vi "Door.vi"() -> ()   [LabVIEW 2011]
uses:
  <vilib>/LabVIEW Interface for Arduino/Type Defs/Board Type.ctl
  <vilib>/LabVIEW Interface for Arduino/Type Defs/Pin Mode.ctl
  <vilib>/LabVIEW Interface for Arduino/LabVIEW Interface for Arduino.lvlib
panel:
  in  "stop 13":bool
  out "Voltage 4":dbl(knob) scale=0.0..5.0
  out "Key Switch open":bool
  out "Numeric":i32
  out "Numeric 2":i32
  out "Door Open":bool
  out "Door Close":bool
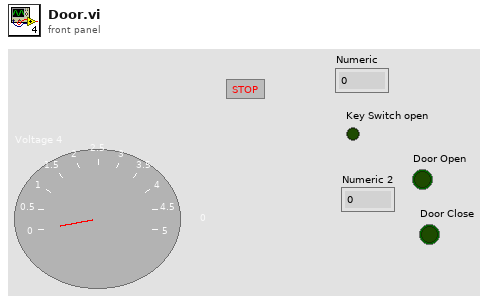
[diagram p1: front panel]
types:
  T1 = typedef "LabVIEW Interface for Arduino.lvlib/Board Type.ctl" = enum16{"Uno", "Dimuelanove w/Atmega 328", "Mega 2560"}
  T2 = typedef "LabVIEW Interface for Arduino.lvlib/Pin Mode.ctl" = enum8{"Input", "Output"}
  T3 = typedef "LabVIEW Interface for Arduino.lvlib/Arduino Resource.ctl" = cluster{"VISA resource":refnum<visa-resource-name>, "Board Type":T1, "Connection Type":enum8{"USB / Serial"}, "Bytes Per Packet (15)":u8}
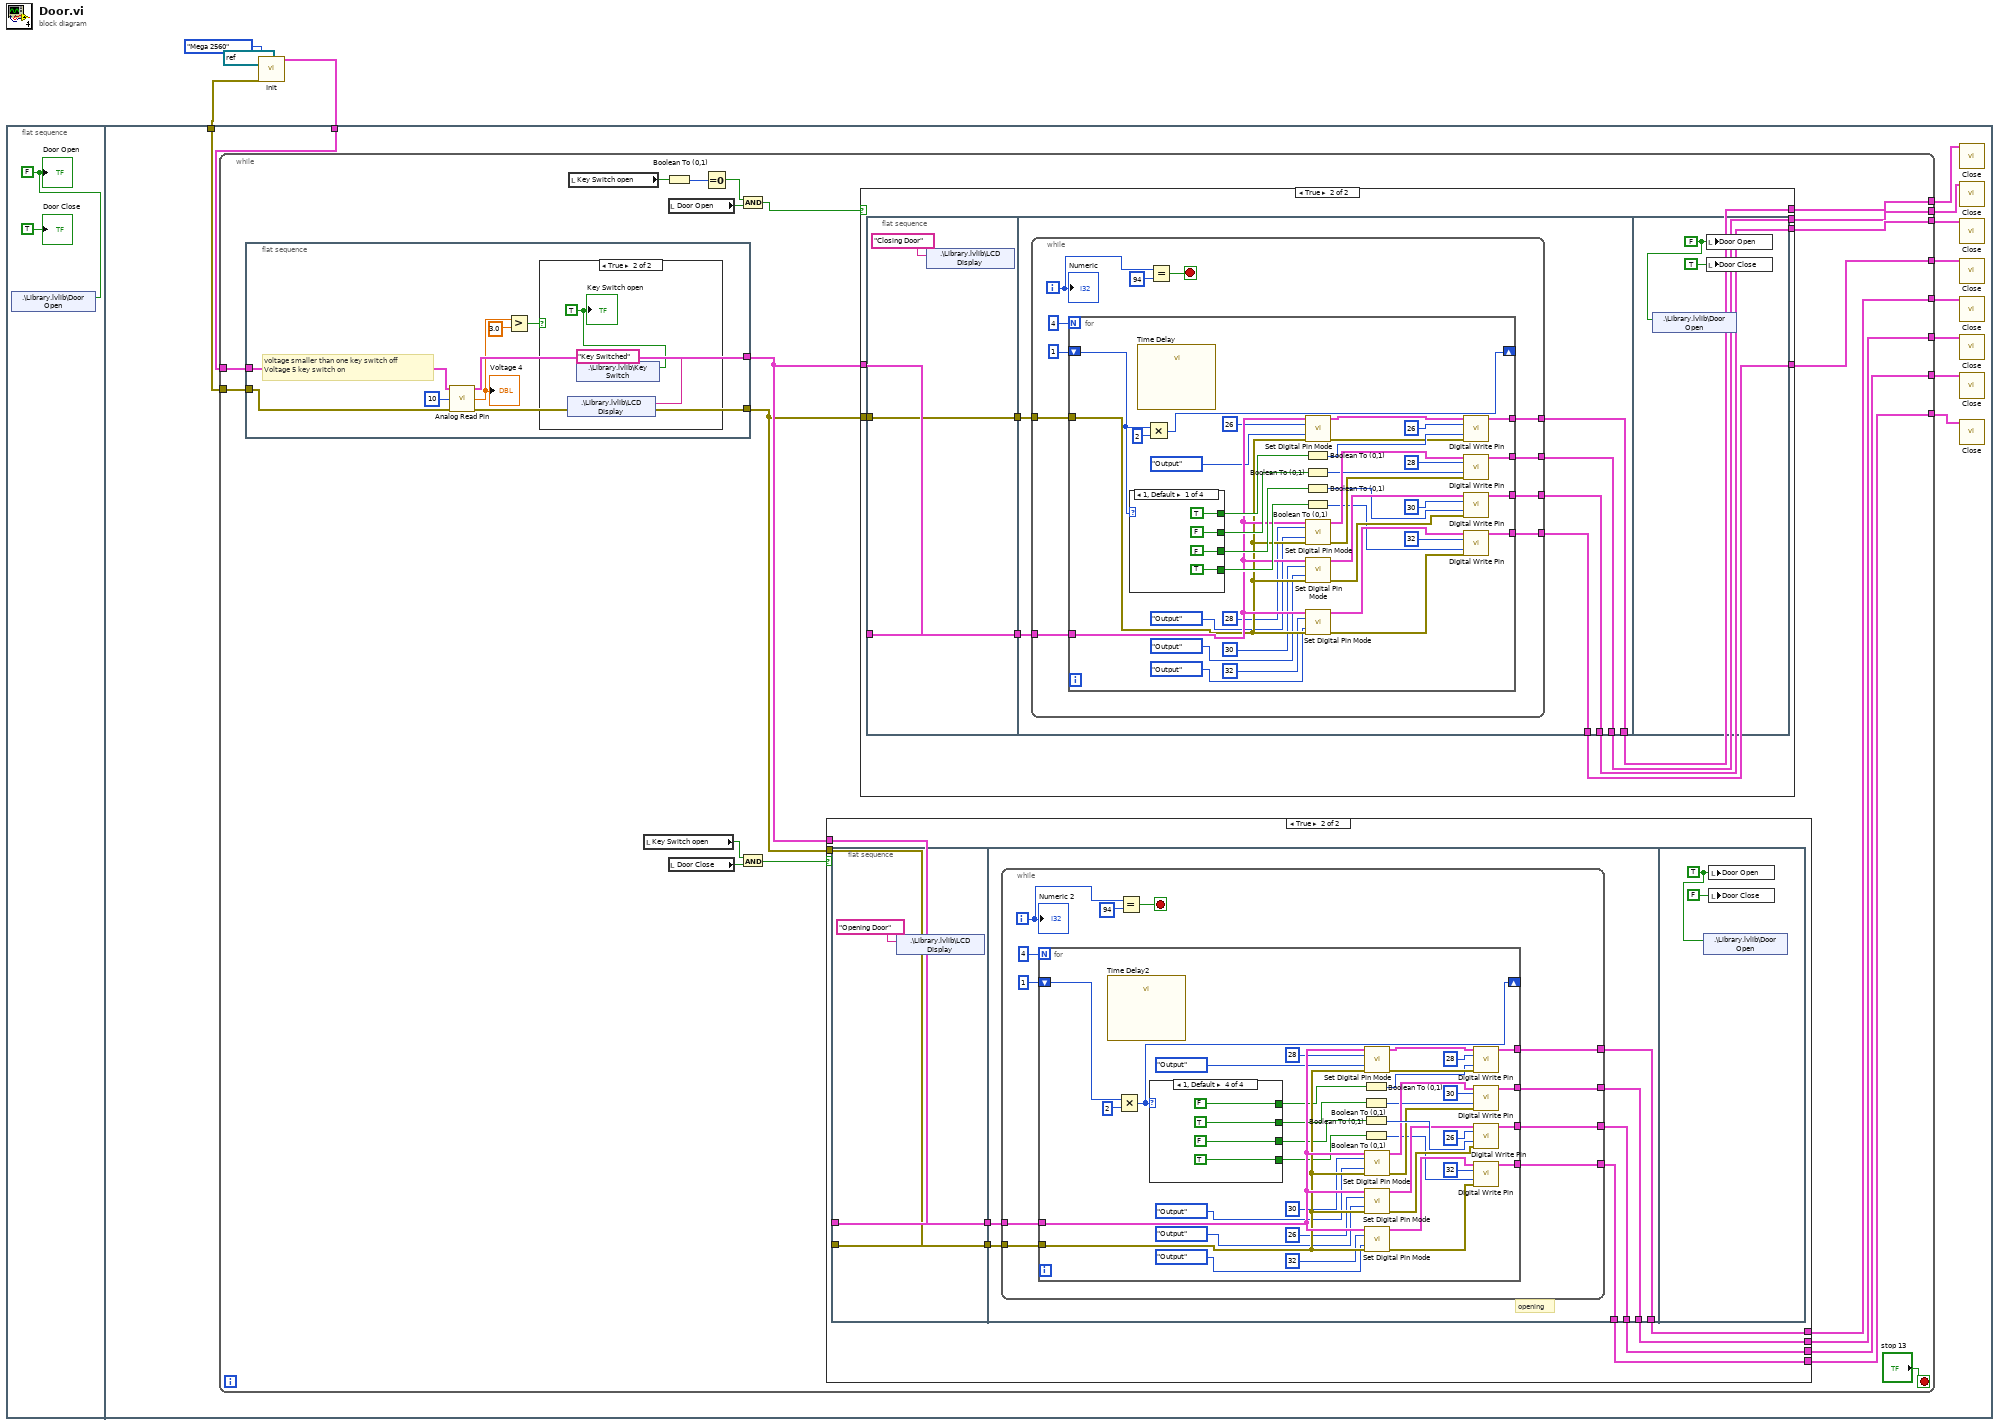
[diagram p0: block diagram]
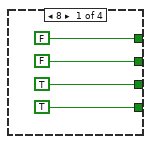
[diagram p3: hidden frame]
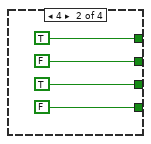
[diagram p4: hidden frame]
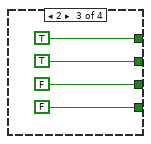
[diagram p5: hidden frame]
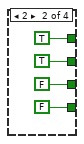
[diagram p7: hidden frame]
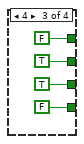
[diagram p8: hidden frame]
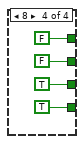
[diagram p9: hidden frame]
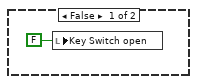
[diagram p10: hidden frame]
diagram:
  n1 = flat-sequence {
    tunnel: w4 -> [w8]
    tunnel: w3 -> [w7]
    frame #0 {
      w5 = FALSE ("Door Open")
      n2 = shared-variable ".\\Library.lvlib\\Door Open"(w5) -> ()  [unwired: 1 in, 1 out]
      "Door Open" <- w5
      "Door Close" <- TRUE ("Door Close")
    }
    frame #1 {
      n3 = while {
        tunnel: w8 -> [w36]
        tunnel: w7 -> [w33]
        tunnel: [w32] -> w16
        tunnel: [w31] -> w15
        tunnel: [w30] -> w14
        tunnel: [w29] -> w13
        tunnel: [w20] -> w12
        tunnel: [w19] -> w11
        tunnel: [w18] -> w10
        tunnel: [w17] -> w9
        stop <- "stop 13" stop-if-true
        n4 = flat-sequence {
          tunnel: w36 -> [w213]
          tunnel: [w211] -> w35
          tunnel: [w210] -> w34
          tunnel: w33 -> [w209]
          frame #0 {
            # "voltage smaller than one key switch off\nVoltage 5 key switch on"
            n5 = call <vilib>:"Analog Read Pin.vi"("Arduino Resource"=w213, "Analog Input Pin (0)"=u8 10, "error in"=w209) -> ("Arduino Resource"=w211:T3, "Voltage"=w208:dbl, "error out"=w210:errorcluster)  [unwired: 10 in]
            "Voltage 4" <- w208
            n6 = Greater?(x=w208, y=3.0) -> (0:w206:bool)
            n7 = case shown="True" w206 {
              frame False {
                n8 = local write "Key Switch open"(FALSE ("Key Switch open")) -> ()
              }
              frame True {
                w216 = TRUE ("Key Switch open")
                n9 = shared-variable ".\\Library.lvlib\\LCD Display"("Key Switched" ("LCD Display")) -> ()  [unwired: 1 in, 1 out]
                n10 = shared-variable ".\\Library.lvlib\\Key Switch"(w216) -> ()  [unwired: 1 in, 1 out]
                "Key Switch open" <- w216
              }
            }
          }
        }
        n11 = local read "Key Switch open"() -> (w24:bool)
        n12 = local read "Key Switch open"() -> (w28:bool)
        n13 = Boolean To (0,1)(Boolean=w24) -> (0, 1=w23:i16)
        n14 = local read "Door Open"() -> (w21:bool)
        n15 = local read "Door Close"() -> (w27:bool)
        n16 = Equal To 0?(x=w23) -> (x = 0?=w22:bool)
        n17 = And(x=w22, y=w21) -> (x .and. y?=w25:bool)
        n18 = And(x=w28, y=w27) -> (x .and. y?=w26:bool)
        n19 = case shown="True" w26 {
          tunnel: w35 -> [w38 w46]
          tunnel: w34 -> [_ w45]
          tunnel: [w38 w44] -> w32
          tunnel: [w38 w43] -> w31
          tunnel: [w38 w42] -> w30
          tunnel: [w38 w41] -> w29
          frame False {
          }
          frame True {
            n20 = flat-sequence {
              tunnel: w45 -> [w48]
              tunnel: w46 -> [w49]
              tunnel: [w49] -> w40
              tunnel: [w48] -> w39
              tunnel: [w53] -> w44
              tunnel: [w52] -> w43
              tunnel: [w51] -> w42
              tunnel: [w50] -> w41
              tunnel: w40 -> [w55]
              tunnel: w39 -> [w54]
              frame #0 {
                n21 = shared-variable ".\\Library.lvlib\\LCD Display"("Opening Door" ("LCD Display")) -> ()  [unwired: 1 in, 1 out]
              }
              frame #1 {
                # "opening"
                n22 = while {
                  tunnel: w55 -> [w64]
                  tunnel: w54 -> [w63]
                  tunnel: [w62] -> w51
                  tunnel: [w61] -> w50
                  tunnel: [w60] -> w53
                  tunnel: [w59] -> w52
                  i -> [w58]
                  stop <- w56 stop-if-true
                  n23 = for {
                    N: 4 -> [_]
                    shift-right: [w67] -> _
                    shift-left: 1 -> [w102]
                    tunnel: w64 -> [w101]
                    tunnel: w63 -> [w100]
                    tunnel: [w75] -> w62
                    tunnel: [w74] -> w61
                    tunnel: [w73] -> w60
                    tunnel: [w72] -> w59
                    n24 = call "Time Delay2"() -> ()  [unwired: 11 in, 1 out]
                    n25 = Multiply(x=w102, y=i8 2) -> (x*y=w67:i32)
                    n26 = case shown="1, Default" w67 {
                      tunnel: [TRUE TRUE FALSE FALSE] -> w68
                      tunnel: [FALSE FALSE TRUE TRUE] -> w70
                      tunnel: [FALSE TRUE TRUE FALSE] -> w71
                      tunnel: [TRUE FALSE FALSE TRUE] -> w69
                      frame 8 {
                      }
                      frame 4 {
                      }
                      frame 2 {
                      }
                      frame 1, Default {
                      }
                    }
                    n27 = Boolean To (0,1)(Boolean=w71) -> (0, 1=w78:i16)
                    n28 = Boolean To (0,1)(Boolean=w70) -> (0, 1=w77:i16)
                    n29 = Boolean To (0,1)(Boolean=w68) -> (0, 1=w99:i16)
                    n30 = Boolean To (0,1)(Boolean=w69) -> (0, 1=w76:i16)
                    n31 = call <vilib>:"Set Digital Pin Mode.vi"("Arduino Resource"=w101, "Digital I/O Pin"=u8 28, "Pin Mode (Input)"=Pin_Mode."Output", "error in"=w100) -> ("Arduino Resource"=w88:T3, "error out"=w87:errorcluster)  [unwired: 10 in]
                    n32 = call <vilib>:"Set Digital Pin Mode.vi"("Arduino Resource"=w101, "Digital I/O Pin"=u8 30, "Pin Mode (Input)"=Pin_Mode."Output", "error in"=w100) -> ("Arduino Resource"=w79:T3, "error out"=w80:errorcluster)  [unwired: 10 in]
                    n33 = call <vilib>:"Set Digital Pin Mode.vi"("Arduino Resource"=w101, "Digital I/O Pin"=u8 26, "Pin Mode (Input)"=Pin_Mode."Output", "error in"=w100) -> ("Arduino Resource"=w89:T3, "error out"=w90:errorcluster)  [unwired: 10 in]
                    n34 = call <vilib>:"Set Digital Pin Mode.vi"("Arduino Resource"=w101, "Digital I/O Pin"=u8 32, "Pin Mode (Input)"=Pin_Mode."Output", "error in"=w100) -> ("Arduino Resource"=w98:T3, "error out"=w97:errorcluster)  [unwired: 10 in]
                    n35 = call <vilib>:"Digital Write Pin.vi"("Arduino Resource"=w88, "Digital I/O Pin (0)"=u8 28, "Value (0)"=w78, "error in"=w87) -> ("Arduino Resource"=w74:T3)  [unwired: 10 in, 1 out]
                    n36 = call <vilib>:"Digital Write Pin.vi"("Arduino Resource"=w79, "Digital I/O Pin (0)"=u8 30, "Value (0)"=w77, "error in"=w80) -> ("Arduino Resource"=w73:T3)  [unwired: 10 in, 1 out]
                    n37 = call <vilib>:"Digital Write Pin.vi"("Arduino Resource"=w89, "Digital I/O Pin (0)"=u8 26, "Value (0)"=w99, "error in"=w90) -> ("Arduino Resource"=w75:T3)  [unwired: 10 in, 1 out]
                    n38 = call <vilib>:"Digital Write Pin.vi"("Arduino Resource"=w98, "Digital I/O Pin (0)"=u8 32, "Value (0)"=w76, "error in"=w97) -> ("Arduino Resource"=w72:T3)  [unwired: 10 in, 1 out]
                  }
                  n39 = Equal?(x=w58, y=94) -> (x = y?=w56:bool)
                  "Numeric 2" <- w58
                }
              }
              frame #2 {
                w120 = TRUE ("Door Open")
                n40 = shared-variable ".\\Library.lvlib\\Door Open"(w120) -> ()  [unwired: 1 in, 1 out]
                n41 = local write "Door Open"(w120) -> ()
                n42 = local write "Door Close"(FALSE ("Door Close")) -> ()
              }
            }
          }
        }
        n43 = case shown="True" w25 {
          tunnel: w35 -> [w122 w130]
          tunnel: w34 -> [_ w129]
          tunnel: [w122 w128] -> w19
          tunnel: [w122 w127] -> w20
          tunnel: [w122 w126] -> w17
          tunnel: [w122 w125] -> w18
          frame False {
          }
          frame True {
            n44 = flat-sequence {
              tunnel: w129 -> [w132]
              tunnel: w130 -> [w133]
              tunnel: [w133] -> w124
              tunnel: [w132] -> w123
              tunnel: [w137] -> w128
              tunnel: [w136] -> w127
              tunnel: [w135] -> w126
              tunnel: [w134] -> w125
              tunnel: w124 -> [w139]
              tunnel: w123 -> [w138]
              frame #0 {
                n45 = shared-variable ".\\Library.lvlib\\LCD Display"("Closing Door" ("LCD Display")) -> ()  [unwired: 1 in, 1 out]
              }
              frame #1 {
                n46 = while {
                  tunnel: w139 -> [w148]
                  tunnel: w138 -> [w147]
                  tunnel: [w146] -> w134
                  tunnel: [w145] -> w135
                  tunnel: [w144] -> w136
                  tunnel: [w143] -> w137
                  i -> [w142]
                  stop <- w140 stop-if-true
                  n47 = for {
                    N: 4 -> [_]
                    shift-right: [w186] -> _
                    shift-left: 1 -> [w185]
                    tunnel: w148 -> [w180]
                    tunnel: w147 -> [w179]
                    tunnel: [w154] -> w146
                    tunnel: [w153] -> w145
                    tunnel: [w152] -> w144
                    tunnel: [w151] -> w143
                    n48 = case shown="1, Default" w185 {
                      tunnel: [TRUE TRUE FALSE FALSE] -> w181
                      tunnel: [FALSE FALSE TRUE TRUE] -> w183
                      tunnel: [FALSE TRUE TRUE FALSE] -> w184
                      tunnel: [TRUE FALSE FALSE TRUE] -> w182
                      frame 1, Default {
                      }
                      frame 2 {
                      }
                      frame 4 {
                      }
                      frame 8 {
                      }
                    }
                    n49 = call "Time Delay"() -> ()  [unwired: 11 in, 1 out]
                    n50 = Multiply(x=w185, y=i8 2) -> (x*y=w186:i32)
                    n51 = Boolean To (0,1)(Boolean=w181) -> (0, 1=w178:i16)
                    n52 = Boolean To (0,1)(Boolean=w184) -> (0, 1=w157:i16)
                    n53 = Boolean To (0,1)(Boolean=w183) -> (0, 1=w156:i16)
                    n54 = Boolean To (0,1)(Boolean=w182) -> (0, 1=w155:i16)
                    n55 = call <vilib>:"Set Digital Pin Mode.vi"("Arduino Resource"=w180, "Digital I/O Pin"=u8 26, "Pin Mode (Input)"=Pin_Mode."Output", "error in"=w179) -> ("Arduino Resource"=w168:T3, "error out"=w169:errorcluster)  [unwired: 10 in]
                    n56 = call <vilib>:"Set Digital Pin Mode.vi"("Arduino Resource"=w180, "Digital I/O Pin"=u8 28, "Pin Mode (Input)"=Pin_Mode."Output", "error in"=w179) -> ("Arduino Resource"=w167:T3, "error out"=w166:errorcluster)  [unwired: 10 in]
                    n57 = call <vilib>:"Set Digital Pin Mode.vi"("Arduino Resource"=w180, "Digital I/O Pin"=u8 30, "Pin Mode (Input)"=Pin_Mode."Output", "error in"=w179) -> ("Arduino Resource"=w158:T3, "error out"=w159:errorcluster)  [unwired: 10 in]
                    n58 = call <vilib>:"Set Digital Pin Mode.vi"("Arduino Resource"=w180, "Digital I/O Pin"=u8 32, "Pin Mode (Input)"=Pin_Mode."Output", "error in"=w179) -> ("Arduino Resource"=w177:T3, "error out"=w176:errorcluster)  [unwired: 10 in]
                    n59 = call <vilib>:"Digital Write Pin.vi"("Arduino Resource"=w168, "Digital I/O Pin (0)"=u8 26, "Value (0)"=w178, "error in"=w169) -> ("Arduino Resource"=w154:T3)  [unwired: 10 in, 1 out]
                    n60 = call <vilib>:"Digital Write Pin.vi"("Arduino Resource"=w167, "Digital I/O Pin (0)"=u8 28, "Value (0)"=w157, "error in"=w166) -> ("Arduino Resource"=w153:T3)  [unwired: 10 in, 1 out]
                    n61 = call <vilib>:"Digital Write Pin.vi"("Arduino Resource"=w158, "Digital I/O Pin (0)"=u8 30, "Value (0)"=w156, "error in"=w159) -> ("Arduino Resource"=w152:T3)  [unwired: 10 in, 1 out]
                    n62 = call <vilib>:"Digital Write Pin.vi"("Arduino Resource"=w177, "Digital I/O Pin (0)"=u8 32, "Value (0)"=w155, "error in"=w176) -> ("Arduino Resource"=w151:T3)  [unwired: 10 in, 1 out]
                  }
                  n63 = Equal?(x=w142, y=94) -> (x = y?=w140:bool)
                  "Numeric" <- w142
                }
              }
              frame #2 {
                w204 = FALSE ("Door Open")
                n64 = shared-variable ".\\Library.lvlib\\Door Open"(w204) -> ()  [unwired: 1 in, 1 out]
                n65 = local write "Door Open"(w204) -> ()
                n66 = local write "Door Close"(TRUE ("Door Close")) -> ()
              }
            }
          }
        }
      }
      n67 = call <vilib>:"Close.vi"("Arduino Resource"=w10) -> ()  [unwired: 14 in, 1 out]
      n68 = call <vilib>:"Close.vi"("Arduino Resource"=w9) -> ()  [unwired: 14 in, 1 out]
      n69 = call <vilib>:"Close.vi"("Arduino Resource"=w12) -> ()  [unwired: 14 in, 1 out]
      n70 = call <vilib>:"Close.vi"("Arduino Resource"=w11) -> ()  [unwired: 14 in, 1 out]
      n71 = call <vilib>:"Close.vi"("Arduino Resource"=w13) -> ()  [unwired: 14 in, 1 out]
      n72 = call <vilib>:"Close.vi"("Arduino Resource"=w16) -> ()  [unwired: 14 in, 1 out]
      n73 = call <vilib>:"Close.vi"("Arduino Resource"=w14) -> ()  [unwired: 14 in, 1 out]
      n74 = call <vilib>:"Close.vi"("Arduino Resource"=w15) -> ()  [unwired: 14 in, 1 out]
    }
  }
  n75 = call <vilib>:"Init.vi"("VISA resource"=refnum<visa-resource-name> "COM4", "Board Type (Uno)"=Board_Type."Mega 2560") -> ("Arduino Resource"=w4:T3, "error out"=w3:errorcluster)  [unwired: 16 in]
